vi "Trinket-LPF2.vi"() -> ()   [LabVIEW 2016]
uses:
  VIs/uPythonX/uPythonX.xctl
panel:
  in  "VISA resource name 2":refnum<visa-resource-name>
  in  "pyboard i2c":T1(xcontrol)={"Port"="Trinket - ASRL108::INSTR", "All Code"="import board,time\nimport busio\nfrom digitalio import DigitalInOut, Direction, Pull\n\ntx = DigitalInOut(board.TX)\ntx.direction = Direction.OUTPUT\ntx.value = 0\ntime.sleep(0.5)\ntx.value = 1\ntx.deinit()\nuart = busio.UART(baudrate=2400, bits=8, parity=None, stop=1,tx = board.TX, rx = board.RX)\nstarttime = time.monotonic()\ncurrenttime = starttime\nwhile (currenttime-starttime) < 2:\n     time.sleep(0.005)\n     data = uart.read(uart.in_waiting)\n     print(data)\n     if data.find(b'\\x04') >= 0:\n          connected = True\n          print(5) \n          currenttime = starttime+3 \n     else:\n          connected = False\n          currenttime = time.monotonic()\n"}
  in  "Trinket i2c":T1(xcontrol)={"Port"="Trinket - ASRL110::INSTR", "All Code"="import board\nfrom i2cslave import I2CSlave\n\nregs = [0] * 16\nindex = 0\n\nwith I2CSlave(board.SCL, board.SDA, (0x40, 0x41)) as slave:\n    while True:\n        r = slave.request()\n        if not r:\n            # Maybe do some housekeeping\n            continue\n        with r:  # Closes the transfer if necessary by sending a NACK or feeding the master dummy bytes\n            if r.address == 0x40:\n                if not r.is_read:  # Master write which is Slave read\n                    b = r.read(1)\n                    if not b or b[0] > 15:\n                        break\n                    index = b[0]\n                    b = r.read(1)\n                    if b:\n                        regs[index] = b[0]\n                elif r.is_restart:  # Combined transfer: This is the Master read message\n                    n = r.write(bytes([regs[index]]))\n                #else:\n                    # A read transfer is not supported in this example\n                    # If the Master tries, it will get 0xff byte(s) by the ctx manager (r.close())\n            elif r.address == 0x41:\n                if not r.is_read:\n                    b = r.read(1)\n                    if b and b[0] == 0xde:\n                        # do something\n                        pass"}
  in  "minimal 2":T2(xcontrol)={"VISA Refnum in"="Trinket - ASRL108::INSTR", "Python Code"="import time as utime\nimport board\nimport busio\nfrom digitalio import DigitalInOut, Direction, Pull\n\nclass LPF2Class:\n     def __init__(self):\n          self.connected = False\n\n     def send_value(self, data):\n          value = (data & 0xFF)\n          payload = bytes([0xC0, value, 0xFF ^ 0xC0 ^ value])\n          size = self.uart.write(payload)\n\n\n     def initialize(self):\n          print(1)\n          tx = DigitalInOut(board.TX)\n          tx.direction = Direction.OUTPUT\n          tx.value = 0\n          utime.sleep(0.5)\n          tx.value = 1\n          tx.deinit()\n          self.uart = busio.UART(baudrate=2400, bits=8, parity=None, stop=1,tx = board.TX, rx = board.RX)\n          self.uart.write(b'\\x00')\n          self.uart.write(b'\\x40\\x23\\x9C')  #CMD_TYPE (x40)  Type   checksum\n          self.uart.write(b'\\x49\\x00\\x00\\xB6')  #CMD_MODE (x49)  # Modes  # Views   checksum\n          self.uart.write(b'\\x52\\x00\\xC2\\x01\\x00\\x6E')  #CMD_SPEED (x52)  baud (LSB first)   checksum\n          self.uart.write(b'\\x5F\\x00\\x00\\x00\\x02\\x00\\x00\\x00\\x02\\xA0')  #CMD_VERSION (x5F)  Hardware_V  Software_V   checksum\n          self.uart.write(b'\\xA0\\x00\\x4C\\x50\\x46\\x32\\x2D\\x44\\x45\\x54\\x45\\x43\\x54\\x00\\x00\\x00\\x00\\x00\\x1D')  #CMD_INFO|bytes|mode  0 name 0   checksum\n          self.uart.write(b'\\x98\\x01\\x00\\x00\\x00\\x00\\x00\\x00\\x20\\x41\\x07')  #CMD_INFO|3|mode  1 (raw) raw_min  raw_max   checksum\n          self.uart.write(b'\\x98\\x02\\x00\\x00\\x00\\x00\\x00\\x00\\xC8\\x42\\xEF')  #CMD_INFO|3|mode  2 (pct) pct_min  pct_max   checksum\n          self.uart.write(b'\\x98\\x03\\x00\\x00\\x00\\x00\\x00\\x00\\x20\\x41\\x05')  #CMD_INFO|3|mode  3 (SI) si_min  si_max   checksum\n          self.uart.write(b'\\x80\\x04\\x00\\x7B')  #CMD_INFO|size|mode  0,4,symbol   checksum\n          self.uart.write(b'\\x88\\x05\\x10\\x00\\x62')  #CMD_INFO|1|mode  5 (FM) Function Map-In   -out   checksum\n          self.uart.write(b'\\x90\\x80\\x01\\x00\\x03\\x00\\xED')  #CMD_INFO|2|mode  x80 sample_size   Data_type   Figures   Decimals   checksum\n          utime.sleep(0.005)\n          self.uart.write(b'\\x04') \n          print(4) \n          starttime = utime.monotonic()\n          currenttime = starttime\n          while (currenttime-starttime) < 2:\n               utime.sleep(0.005)\n               data = self.uart.read(self.uart.in_waiting)\n               print(data)\n               if data.find(b'\\x04') >= 0:\n                    self.connected = True\n                    print(5) \n                    currenttime = starttime+3 \n               else:\n                    self.connected = False\n                    currenttime = utime.monotonic()\n          \n          self.uart.deinit()\n          tx = DigitalInOut(board.TX)\n          tx.direction = Direction.OUTPUT\n          tx.value = 0\n          utime.sleep(0.01)\n          tx.deinit()\n          self.uart = busio.UART(baudrate=115200, bits=8, parity=None, stop=1,tx = board.TX, rx = board.RX)\n          self.send_value(2)\ni = 0\nlpf2 = LPF2Class()\nlpf2.initialize()\nprint(lpf2.connected)\n\nwhile lpf2.connected:\n    lpf2.send_value(i)\n    i += 1\n    if i > 10: \n        i = 0\n    utime.sleep(0.2)\n          "}
  in  "VISA resource name":refnum<visa-resource-name>
  in  "microbit":T2(xcontrol)={"VISA Refnum in"="ASRL108::INSTR", "Python Code"="import time as utime\nimport gc\nfrom microbit import *\n\nclass LPF2Class:\n    def __init__(self):\n        self.connected = False\n        self.tx = pin0\n        self.rx = pin1\n        self.watchdog = 0\n\n    def init_uart(self,baud):\n        return uart.init(baudrate=baud, bits=8, parity=None, stop=1,tx = self.tx, rx = self.rx)\n    def write_uart(data):\n        if len(data) > 1:\n            for b in array:\n                chksm ^= b\n            chksm ^= 0xFF\n            data.append(chksm)\n        return self.uart.write(bytes(data))\n    def read_uart(self):\n        return uart.read(uart.any())\n    def close_uart(self):\n        return self.uart.deinit()\n    def pulse_tx(self,value):\n        return self.tx.write_digital(value)\n    def get_time(self):\n        return utime.ticks_ms() / 1000\n\n    "}
  in  "minimal":T2(xcontrol)={"VISA Refnum in"="Trinket - ASRL110::INSTR", "Python Code"="import time as utime\nimport board\nimport busio\nfrom digitalio import DigitalInOut, Direction, Pull\n\nclass LPF2Class:\n     def __init__(self):\n          self.connected = False\n          self.watchdog = 0\n          \n     def init_uart(self,baud):\n          self.uart = busio.UART(baudrate=baud, bits=8, parity=None, stop=1,tx = board.TX, rx = board.RX)\n\n     def write_uart(self,data):\n          chksm = 0xFF\n          if len(data) > 1:\n               for b in data:\n                    chksm ^= b\n               data.append(chksm)\n          return self.uart.write(bytes(data))\n          \n     def read_uart(self):\n          return self.uart.read(self.uart.in_waiting)\n          \n     def close_uart(self):\n          return self.uart.deinit()\n          \n     def init_tx(self):\n          self.tx = DigitalInOut(board.TX)\n          self.tx.direction = Direction.OUTPUT\n \n     def pulse_tx(self,start_value,time,stop_value):\n          self.tx = DigitalInOut(board.TX)\n          self.tx.direction = Direction.OUTPUT\n          self.tx.value = start_value\n          utime.sleep(time)\n          self.tx.value = stop_value\n          self.tx.deinit()\n                              \n     def get_time(self):\n          return utime.monotonic()\n\n     def send_value(self, data):\n          size = self.write_uart([0xC0,data & 0xFF])\n          if not size:\n               self.connected = False\n               \n     def read_value(self):\n          data = self.read_uart()\n          if len(data) > 0:\n               self.watchdog = self.get_time()\n          self.coonnected = (self.get_time() - self.watchdog) < 2\n          return data\n     \n     def reset(self):\n          self.pulse_tx(0, 0.5, 1)\n          self.init_uart(2400)\n          self.write_uart([0])\n          self.write_uart([0x40,35])  #CMD_TYPE (x40)  Type   checksum\n          self.write_uart([0x49,0,0])  #CMD_MODE (x49)  # Modes  # Views   checksum\n          self.write_uart([0x52,0,0xC2,1,0])  #CMD_SPEED (x52)  baud (LSB first)   checksum\n          self.write_uart([0x5F,0,0,0,2,0,0,0,2])  #CMD_VERSION (x5F)  Hardware_V  Software_V   checksum\n          Name = [0xA0,0] + [x for x in b'LPF2-DETECT'] + [0,0,0,0,0] #CMD_INFO|bytes|mode  0 name 0   checksum\n          self.write_uart(Name) \n          self.write_uart([0x98,1,0,0,0,0,0,0,32,65])  #CMD_INFO|3|mode  1 (raw) raw_min  raw_max   checksum\n          self.write_uart([0x98,2,0,0,0,0,0,0,200,66])  #CMD_INFO|3|mode  2 (pct) pct_min  pct_max   checksum\n          self.write_uart([0x98,3,0,0,0,0,0,0,32,65])  #CMD_INFO|3|mode  3 (SI) si_min  si_max   checksum\n          self.write_uart([0x80,4,0])  #CMD_INFO|size|mode  0,4,symbol   checksum\n          self.write_uart([0x88,5,16,0])  #CMD_INFO|1|mode  5 (FM) Function Map-In   -out   checksum\n          self.write_uart([0x90,0x80,1,0,3,0])  #CMD_INFO|2|mode  x80 sample_size   Data_type   Figures   Decimals   checksum\n          utime.sleep(0.005)\n          self.write_uart([4])   #ACK\n          starttime = self.get_time()\n          currenttime = starttime\n          while (currenttime-starttime) < 2:\n               utime.sleep(0.005)\n               data = self.read_value()\n               print(data)\n               if data.find(b'\\x04') >= 0:\n                    self.connected = True\n                    self.close_uart()\n                    self.pulse_tx(0,0.01,0)\n                    self.init_uart(115200)\n                    self.watchdog = self.get_time()\n                    self.send_value(2)\n                    currenttime = starttime + 2\n               else:\n                    self.connected = False\n                    currenttime = self.get_time()\n          \n\ni = 0\nlpf2 = LPF2Class()\nlpf2.reset()\nprint('Success' if lpf2.connected else 'Falied')\n'''\nwhile True:\n     if lpf2.connected:\n          lpf2.send_value(i)\n          lpf2.read_value()\n          i += 1 if i < 9 else -9\n          utime.sleep(0.2)\n     else:\n          print('trying')\n          lpf2.reset()\n'''\n\n"}
  in  "LPF2Class.py":T2(xcontrol)={"VISA Refnum in"="PyBoard - ASRL104::INSTR", "Python Code"="import time as utime\nimport board\nimport busio\nfrom digitalio import DigitalInOut, Direction, Pull\n\nCMD_Type = 0x40   # set sensor type command\nCMD_Mode = 0x49   # set mode type command\nCMD_Baud = 0x52   # set the transmission baud rate\nCMD_Vers = 0x5F   # set the version number\nCMD_ModeInfo = 0x80  # name command\n\nNAME,RAW,Pct,SI,SYM,FCT, FMT = 0x0,0x1,0x2,0x3,0x4,0x5, 0x80\nDATA8,DATA16,DATA32,DATAF = 0,1,2,3  # Data type codes\nABSOLUTE,RELATIVE,DISCRETE = 16,8,4\n\n# Name, Format [# datasets, type, figures, decimals], raw [min,max], Percent, SI, Symbol,functionMap, view\nmode0 = ['LPF2-DETECT',[1,DATA8,3,0],[0,10],[0,100],[0,10],'',[ABSOLUTE,0],True]\nmode1 = ['LPF2-COUNT',[1,DATA32,4,0],[0,100],[0,100],[0,100],'CNT',[ABSOLUTE,0],True]\nmode2 = ['LPF2-CAL',[3,DATA16,3,0],[0,1023],[0,100],[0,1023],'RAW',[ABSOLUTE,0],False]\nmodes = [mode0,mode1,mode2]\n\nclass LPF2(object):\n     def __init__(self):\n          self.connected = False\n          self.payload = bytearray([])\n          self.oldbuffer =  bytes([])\n\n     def load_payload(self,data):\n          value = (data & 0xFF)\n          self.payload = bytes([0xC0, value, 0xFF ^ 0xC0 ^ value])\n          \n     def sendCall(self, timerInfo):\n          if self.connected:\n               size = self.writeIt(self.payload)\n               if not size: self.connected = False\n\n     def writeIt(self,array):\n          #print(binascii.hexlify(array))\n          return self.uart.write(array)\n\n     def readIt(self, timeout = 2):\n          starttime = utime.time()\n          payload = b'\\x02'\n          while (utime.time()-starttime) < timeout:\n               utime.sleep(0.001)\n               if self.uart.in_waiting <6:\n                    continue\n               char = self.uart.read(1)[0]\n               if not (char == ord(b'F')):\n                    continue\n               char = self.uart.read(1)[0]\n               if not (char == ord(b'\\x00')):\n                    continue\n               char = self.uart.read(1)[0]\n               if not (char == ord(b'\\xb9')):\n                    continue\n               char = self.uart.read(1)[0]\n               size = 2**((char & 0b111000)>>3)\n               mode = char & 0b111\n               while (self.uart.in_waiting < size+1):\n                    if (utime.time()-starttime) > timeout:\n                         return payload\n                    utime.sleep(0.01)   # wait for all bytes to come in\n               payload = self.uart.read(size)\n               chksm = self.uart.read(1)[0]\n               calc_chksm = 0xFF ^ char\n               for i in payload:\n                    calc_chksm ^= i\n               print(payload,chksm,calc_chksm,size,mode)\n          return payload\n\n     def waitFor (self, char, timeout = 2):\n          starttime = utime.monotonic()\n          currenttime = starttime\n          status = False\n          while (currenttime-starttime) < timeout:\n               utime.sleep(0.005)\n               currenttime = utime.monotonic()\n               if self.uart.in_waiting > 0:\n                    data = self.uart.read(1)[0]\n                    if  data == ord(char):\n                         status = True\n                         break\n          return status\n\n     def addChksm(self,array):\n          chksm = 0\n          for b in array:\n               chksm ^= b\n          chksm ^= 0xFF\n          array.append(chksm)  \n          return array\n          \n     def init(self):\n          tx = DigitalInOut(board.TX)\n          tx.direction = Direction.OUTPUT\n          tx.value = 0\n          utime.sleep(0.5)\n          tx.value = 1\n          tx.deinit()\n          \n          self.uart= busio.UART(baudrate=2400, bits=8, parity=None, stop=1)\n          self.writeIt(b'\\x00')\n\n     def type(self,sensorType):\n          return self.addChksm(bytearray([CMD_Type, sensorType]))\n\n     def defineBaud(self,baud):\n          rate = baud.to_bytes(4, 'little')\n          return self.addChksm(bytearray([CMD_Baud]) + rate) \n\n     def defineVers(self,hardware,software):\n          hard = hardware.to_bytes(4, 'big')\n          soft = software.to_bytes(4, 'big')\n          return self.addChksm(bytearray([CMD_Vers]) + hard + soft)\n          \n     def padString(self,string, num, startNum):\n          reply = bytearray([startNum])  # start with name\n          reply += string\n          exp = math.ceil(math.log(len(string),2)) if len(string)>0 else 0  # find the next power of 2\n          size = 2**exp\n          exp = exp<<3\n          length = size - len(string)\n          for i in range(length):\n               reply += bytearray([0])\n          return self.addChksm(bytearray([CMD_ModeInfo | exp | num]) + reply)\n\n     def buildFunctMap(self,mode, num, Type):\n          exp = 1 << 3\n          mapType = mode[0]\n          mapOut = mode[1]\n          return self.addChksm(bytearray([CMD_ModeInfo | exp | num, Type, mapType, mapOut]))\n\n     def buildFormat(self,mode, num, Type):\n          exp = 2 << 3\n          sampleSize = mode[0] & 0xFF\n          dataType = mode[1] & 0xFF\n          figures = mode[2] & 0xFF\n          decimals = mode[3] & 0xFF\n          return self.addChksm(bytearray([CMD_ModeInfo | exp | num, Type, sampleSize, dataType,figures,decimals]))\n     \n     def buildRange(self,settings, num, rangeType):\n          exp = 3 << 3\n          minVal = struct.pack('<f', settings[0])\n          maxVal = struct.pack('<f', settings[1])\n          return self.addChksm(bytearray([CMD_ModeInfo | exp | num, rangeType]) + minVal + maxVal)\n\n     def defineModes(self,modes):\n          length = (len(modes)-1) & 0xFF\n          views = 0\n          for i in modes:\n               if (i[7]):\n                    views = views + 1\n          views = (views - 1) & 0xFF\n          return self.addChksm(bytearray([CMD_Mode, length, views]))\n          \n     def setupMode(self,mode,num):\n          self.writeIt(self.padString(mode[0],num,NAME)) # write name\n          self.writeIt(self.buildRange(mode[2], num, RAW)) # write RAW range\n          self.writeIt(self.buildRange(mode[3], num, Pct)) # write Percent range\n          self.writeIt(self.buildRange(mode[4], num, SI)) # write SI range\n          self.writeIt(self.padString(mode[5],num,SYM)) # write symbol\n          self.writeIt(self.buildFunctMap(mode[6],num, FCT)) # write Function Map\n          self.writeIt(self.buildFormat(mode[1],num, FMT)) # write format\n\n     def initialize(self):\n          self.connected = False\n          self.init()\n          self.writeIt(self.type(35))  # set type to 35 \n          self.writeIt(self.defineModes(modes))  # tell how many modes \n          self.writeIt(self.defineBaud(115200))\n          self.writeIt(self.defineVers(2,2))\n\n          num = len(modes) - 1\n          for mode in reversed(modes):\n               self.setupMode(mode,num)\n               num -= 1\n               utime.sleep(0.005)\n               \n          self.writeIt(b'\\x04')  #ACK\n          # Check for ACK reply\n          self.connected = self.waitFor(b'\\x04')\n          print('Success' if self.connected else 'Failed')\n\n          # Reset Serial to High Speed\n          # pull pin low\n          self.uart.deinit()\n          if self.connected:\n               tx = DigitalInOut(board.TX)\n               tx.direction = Direction.OUTPUT\n               tx.value = 0\n               utime.sleep(0.01)\n               tx.deinit()\n               #change baudrate\n               self.uart=busio.UART(baudrate=115200, bits=8, parity=None, stop=1)\n               self.load_payload(2)\n          \n          return\n          \nlpf2 = LPF2()\nlpf2.initialize()\n"}
  in  "Spike":T2(xcontrol)={"VISA Refnum in"="Spike - ASRL73::INSTR", "Python Code"="import hub,utime\n\nhub.port.B.info()\n\n# if info comes back with None - then you have to restart the pybaord\ni=0\nfred = bytes([11])\nwhile (i<15):\n     try:\n          i=i+1 if i<19 else 10\n          value = hub.port.B.device.get()[0]\n          #print(value)\n          hub.display.show(str(value))\n          #print(value)\n          hub.port.B.device.mode(0,fred*i)\n          utime.sleep(0.1)\n     except:\n          utime.sleep(1)\n     \n\n'''\nhub.port.B.device.mode([(0,0),(1,0),(1,2),(3,0)])\n\nhub.port.B.device.mode(0,b'hi there')\n'''"}
  in  "Camera":T2(xcontrol)={"VISA Refnum in"="PyBoard - ASRL104::INSTR", "Python Code"="import gc,utime\nimport pyb, micropython\nfrom LPF2Class import LPF2\n\nmicropython.alloc_emergency_exception_buf(200)\n\nred_led=pyb.LED(1)\ngreen_led = pyb.LED(2)\nred_led.on()\n\n#lpf2 = LPF2(3, 'P4', 'P5', timer = 4, freq = 5)    # OpenMV\nlpf2 = LPF2(1, 'Y1', 'Y2', timer = 4, freq = 5)    # PyBoard\nlpf2.initialize()\n\nvalue = 0\n\n# Loop\nwhile True:\n     if not lpf2.connected:\n          lpf2.sendTimer.callback(None)\n          red_led.on()\n          utime.sleep_ms(200)\n          lpf2.initialize()\n     else:\n          red_led.off()\n          value = value + 1 if value < 9 else 0\n          lpf2.load_payload(value)\n          data = lpf2.readIt()\n          utime.sleep_ms(10)\n          if len(data) > 1:\n               print(data)\n               if data.find(b'toggle')>=0:\n                    green_led.toggle()\n\n          utime.sleep_ms(90)\n\n"}
  # "Download this to your backpack"
  # "Run this on SPIKE\n(and close the window)"
  # "Edit this code"
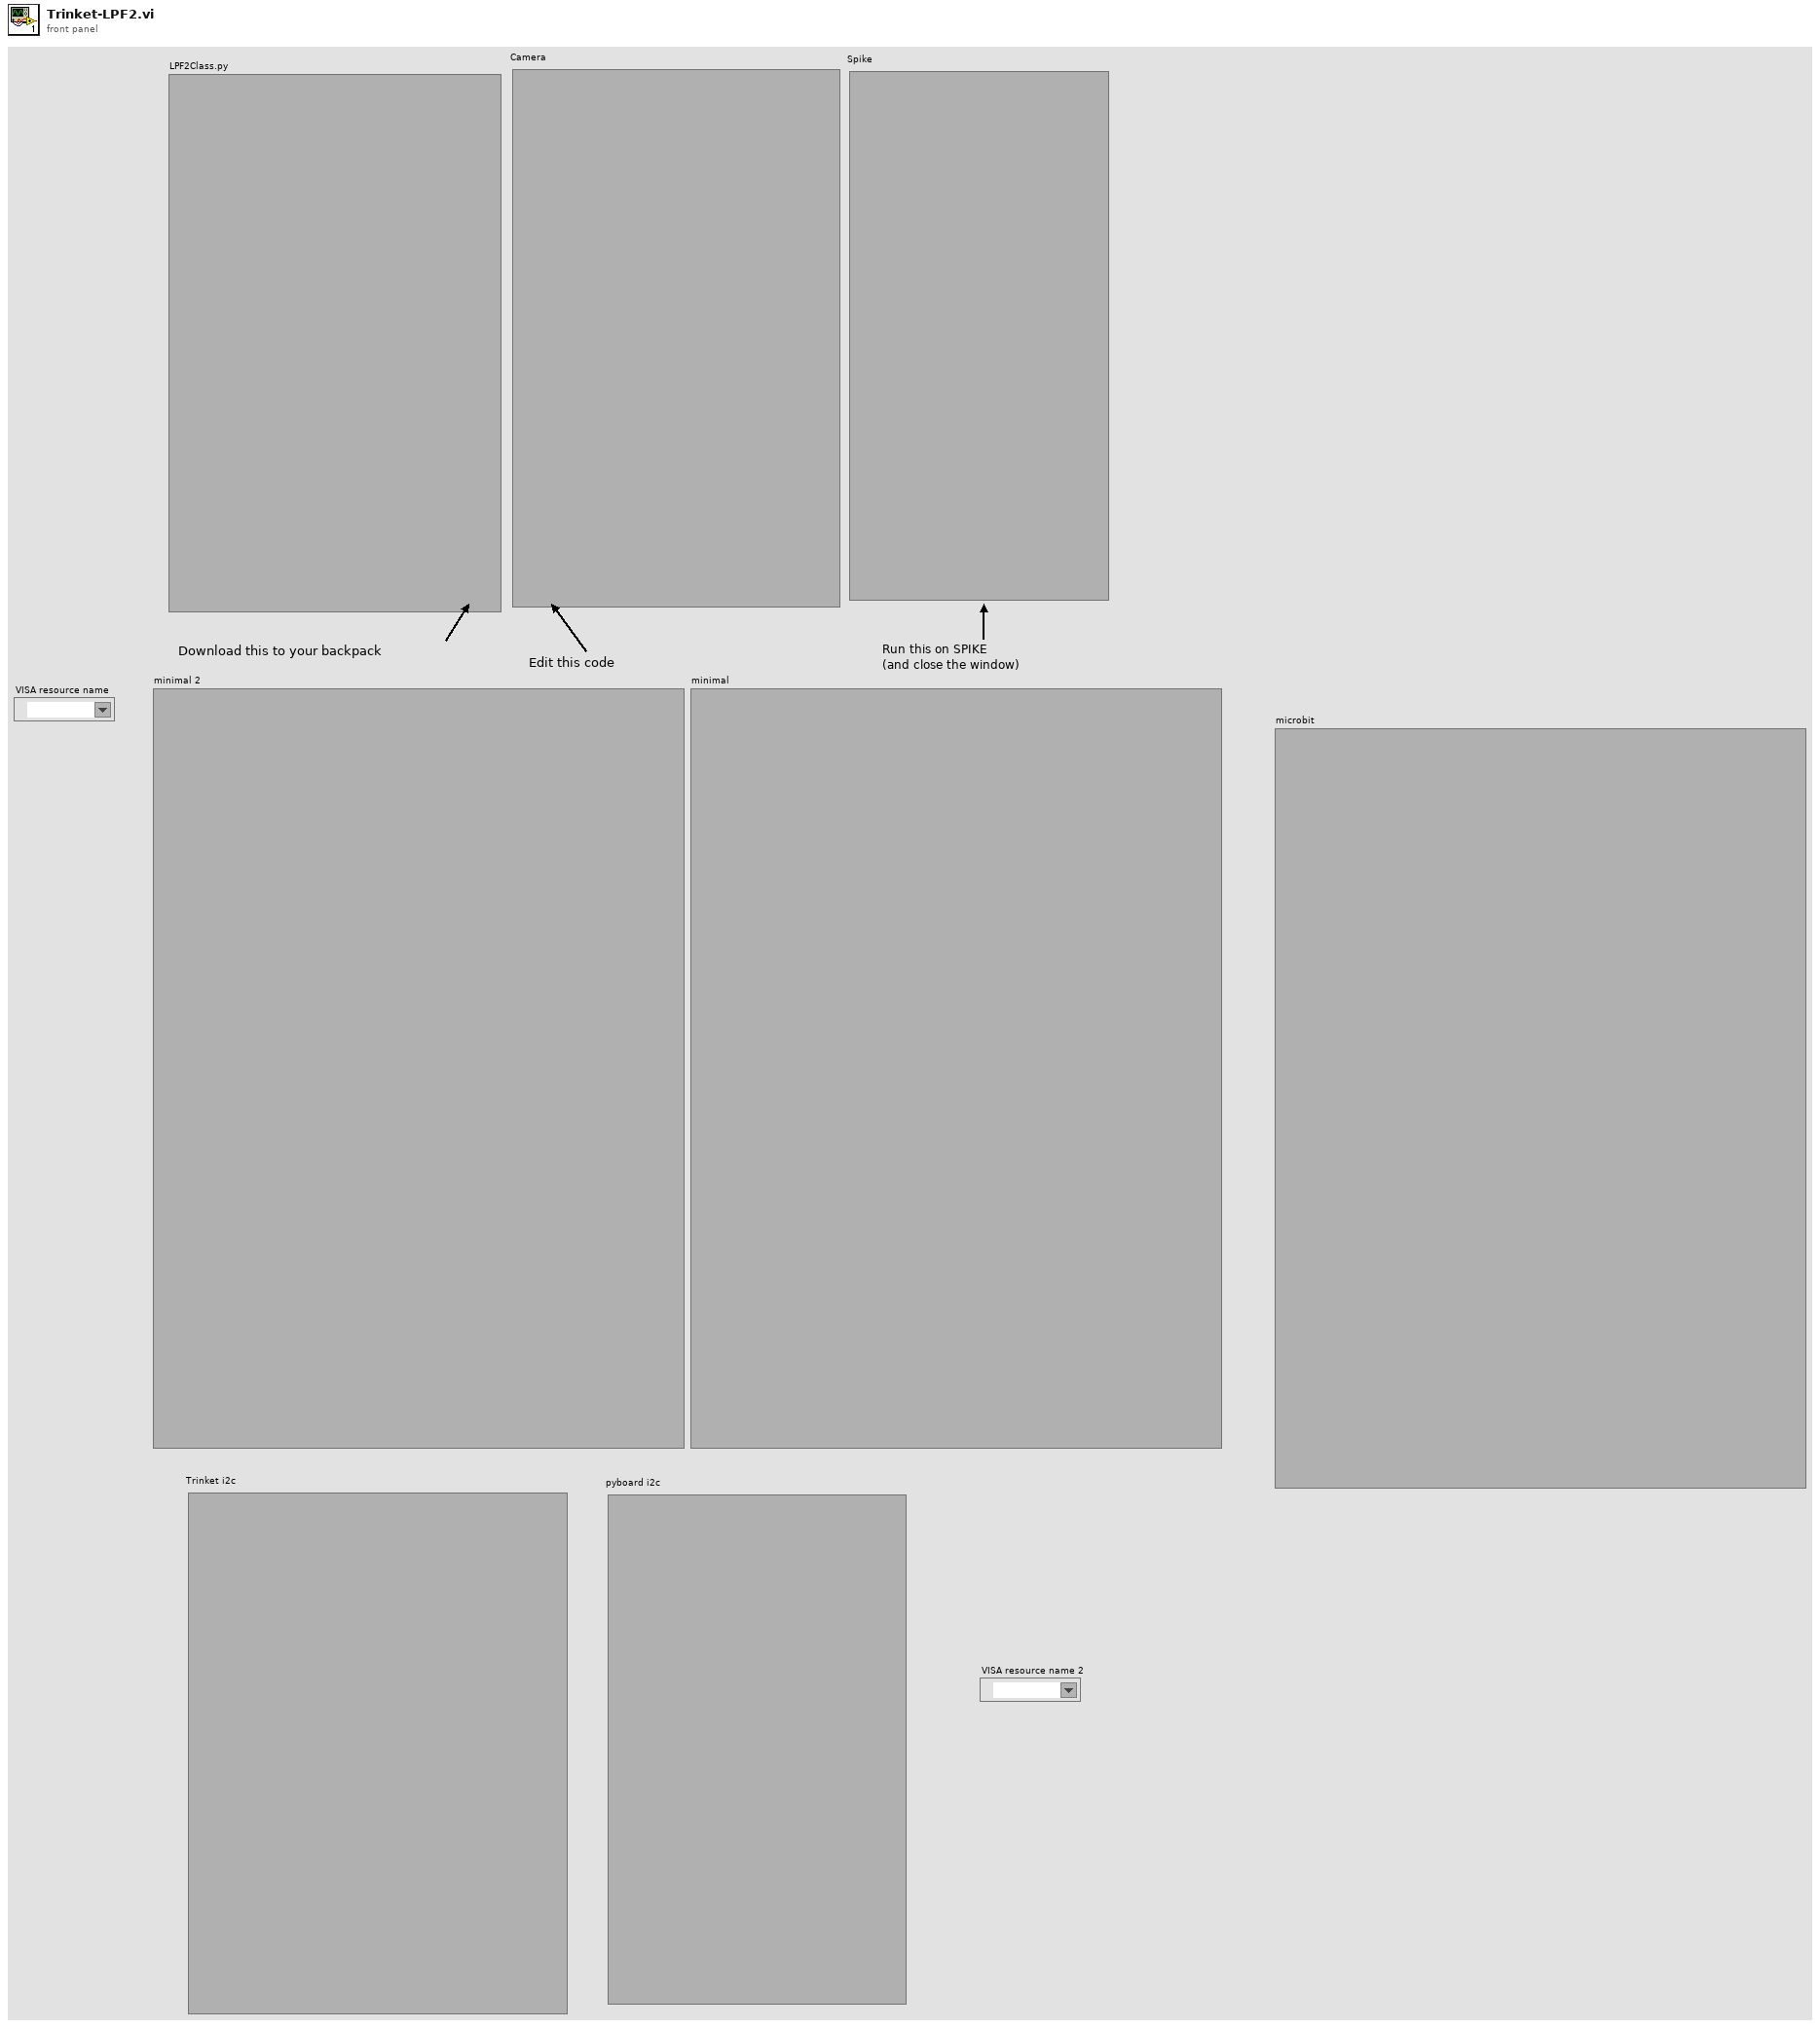
[diagram p1: front panel]
types:
  T1 = cluster{"Port":refnum<visa-resource-name>, "All Code":string}
  T2 = cluster{"VISA Refnum in":refnum<visa-resource-name>, "Python Code":string}
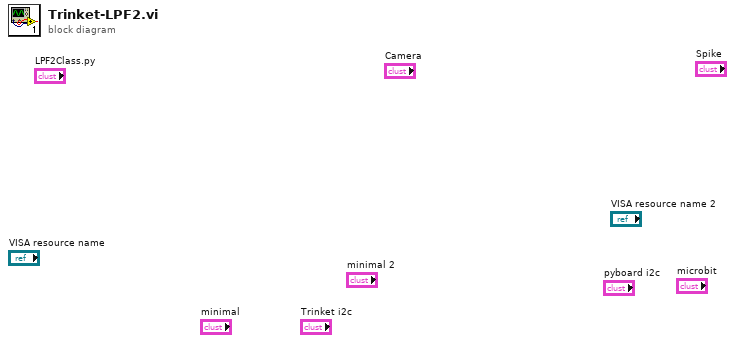
[diagram p0: block diagram]
diagram:
